vi "DSF.Engine.Sequencer Bundle.Get Plugin Timing.vi"(8 "error in (no error)":errorcluster, 11 "Sequencer Bundle in":refnum<class "DSF.Engine.Sequencer Bundle.lvclass">) -> (0 "error out":errorcluster, 2 "Plugin Timing":refnum<class "DSF.Shared.Timing.lvclass">, 3 "Sequencer Bundle out":refnum<class "DSF.Engine.Sequencer Bundle.lvclass">)   [LabVIEW 2016, in "DSF.Engine.lvlib" / "DSF.Engine.Sequencer Bundle.lvclass"]
uses:
  DSF.Engine.Sequencer Bundle.lvclass
  Shared/Classes/Timing/DSF.Shared.Timing.lvclass
  DSF.Engine.Sequencer Bundle.lvclass/DSF.Engine.Sequencer Bundle.ctl
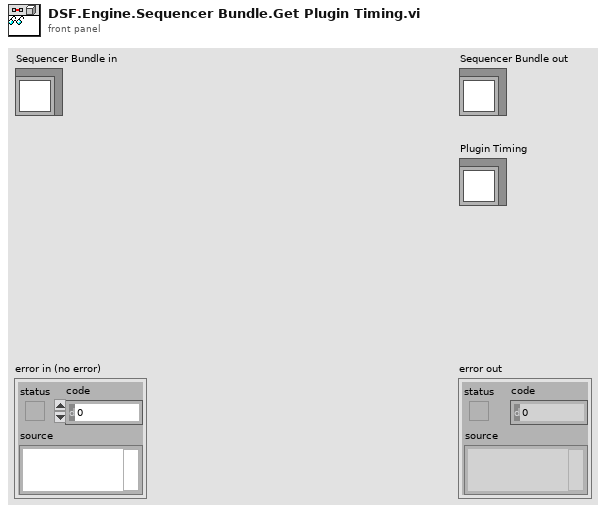
[diagram p1: front panel]
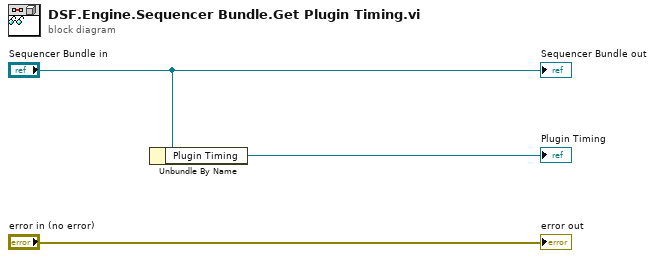
[diagram p0: block diagram]
diagram:
  n1 = Unbundle By Name("Sequencer Bundle in") -> ("Plugin Timing"=→"Plugin Timing":refnum<class "DSF.Shared.Timing.lvclass">)
  "error out" <- "error in (no error)"
  "Sequencer Bundle out" <- "Sequencer Bundle in"
